vi "Read Payload bytes.vi"(8 "error in (no error)":errorcluster, 11 "MsgPackExt in":refnum<class "MsgPackExt.lvclass">) -> (0 "error out":errorcluster, 2 "Payload bytes":u8[](array[numeric]) format="%x", 3 "MsgPackExt out":refnum<class "MsgPackExt.lvclass">)   [LabVIEW 2020, in "MessagePack.lvlib" / "MsgPackExt.lvclass"]
uses:
  MsgPackExt.lvclass
  MsgPackExt.lvclass/MsgPackExt.ctl
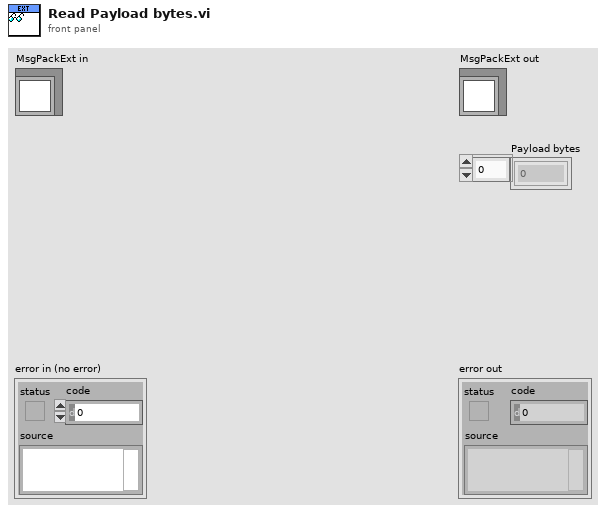
[diagram p1: front panel]
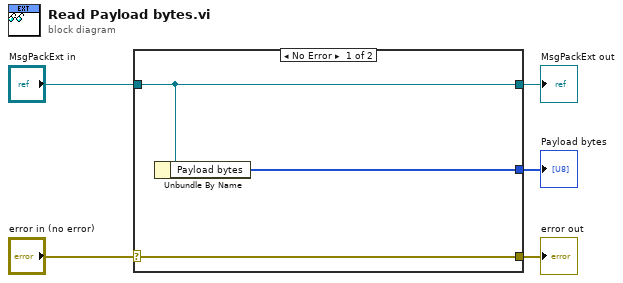
[diagram p0: block diagram]
diagram:
  n1 = case shown="No Error" "error in (no error)" {
    selector: "error in (no error)" -> [w8 w9]
    tunnel: [w8 w9] -> w4
    tunnel: [w7 w10] -> w2
    tunnel: "MsgPackExt in" -> [w7 w10]
    tunnel: [w6 _] -> w1
    frame No Error {
      n2 = Unbundle By Name(w7) -> ("Payload bytes"=w6:u8[])
    }
    frame Error {
    }
  }
  "error out" <- w4
  "MsgPackExt out" <- w2
  "Payload bytes" <- w1
